vi "TestInformation.vi"(7 "LabVIEW Web Service Request":refnum<class "Web Request.lvclass">) -> ()   [LabVIEW 2014]
uses:
  <vilib>/wsapi/Web Request.lvclass
  Coding Platform.lvlib
panel:
  # "Use the Web Service Request input terminal to call the VIs on the Web Services palette. Do not remove it from the connector pane unless you don't need access to the palette."
  # "Each additional control wired to the connector pane will be available as an input in the URL. To include an indicator in terminal-mode output (the default setting), it must also be wired to the connector pane."
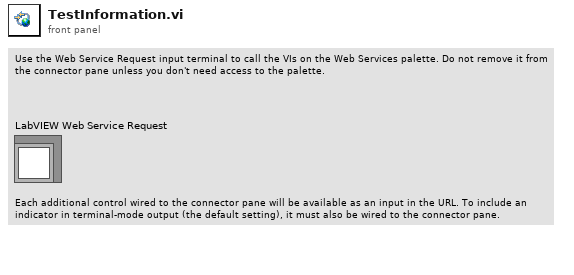
[diagram p1: front panel]
types:
  T1 = typedef "Coding Platform.lvlib/Test Description.ctl" = cluster{"TestName":string, "Description":string, "Status":string, "cID":string[], "qID":string[]}
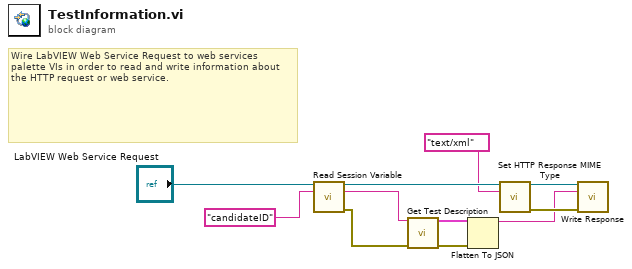
[diagram p0: block diagram]
diagram:
  # "Wire LabVIEW Web Service Request to web services palette VIs in order to read and write information about the HTTP request or web service."
  n1 = call <vilib>:"Read Session Variable.vi"("LabVIEW Web Service Request"="LabVIEW Web Service Request", "key"="candidateID") -> ("LabVIEW Web Service Request out"=w7:refnum<class "Web Request.lvclass">, "value"=w9:string, "error out"=w10:errorcluster)  [unwired: 11 in]
  n2 = call "Get Test Description.vi"("Candidate ID"=w9, "error in (no error)"=w10) -> ("Test Description"=w8:T1, "error out"=w6:errorcluster)  [unwired: 12 in]
  n3 = Flatten To JSON(anything=w8, error in (no error)=w6) -> (JSON string=w1:string)  [unwired: 1 in, 1 out]
  n4 = call <vilib>:"Set HTTP Response MIME Type.vi"("LabVIEW Web Service Request"=w7, "MIME type (text/html)"="text/xml") -> ("LabVIEW Web Service Request out"=w5:refnum<class "Web Request.lvclass">, "error out"=w3:errorcluster)  [unwired: 12 in]
  n5 = call <vilib>:"Write Response.vi"("LabVIEW Web Service Request"=w5, "response string"=w1, "error in (no error)"=w3) -> ()  [unwired: 11 in, 2 out]
